vi "Broadcast D-O Settings.vi"(8 "error in (no error)":errorcluster, 10 "Message Queues":T7, 11 "D-O Module Config":T1={"GUID"="", "Drop Coords"={"Horizontal"=0, "Vertical"=0}, "Process Name"="", "User name"="", "Queue Name"="", "Settings"={"Valve Settings"={"D-O Settings"={"DAQmx Task Name"="", "Output Channel"=0, "Output Channel Names"=[]}, "VICI Electronic Actuator"={"VISA resource name"="", "Mode"=enum."Two Positions With Stops", "Simulated"=FALSE}}, "Valve Type"=enum."Digital Output Valve", "Time On (Sec)"=0.0, "Time Off (Sec)"=0.0, "Run?"=FALSE}, "Load Count"=0} {"Settings"."Valve Settings"."D-O Settings"."Output Channel" items=["Choose a Channel"]}) -> (0 "error out":errorcluster)   [LabVIEW 2018, in "D-O Module.lvlib"]
uses:
  D-O Module.lvlib
  All Message Queues.ctl
  support/Message Queue/Message Cluster.ctl
  D-O Module Config Cluster.ctl
  <vilib>/Utility/miscctls.llb/LVPoint32TypeDef.ctl
  Valve Clusters.ctl
  D-O Module Settings Cluster.ctl
  D-O Device Settings Cluster.ctl
  VICI Electronic Actuator/VICI Electronic Actuator Settings.ctl
  support/Message Queue/Enqueue Message (Single).vi
  support/Message Queue/Message Queue.lvlib
  Shared Variables/Dynamic Shared Variables.lvlib
  DIO Valve/VICI Electronic Actuator.lvlib
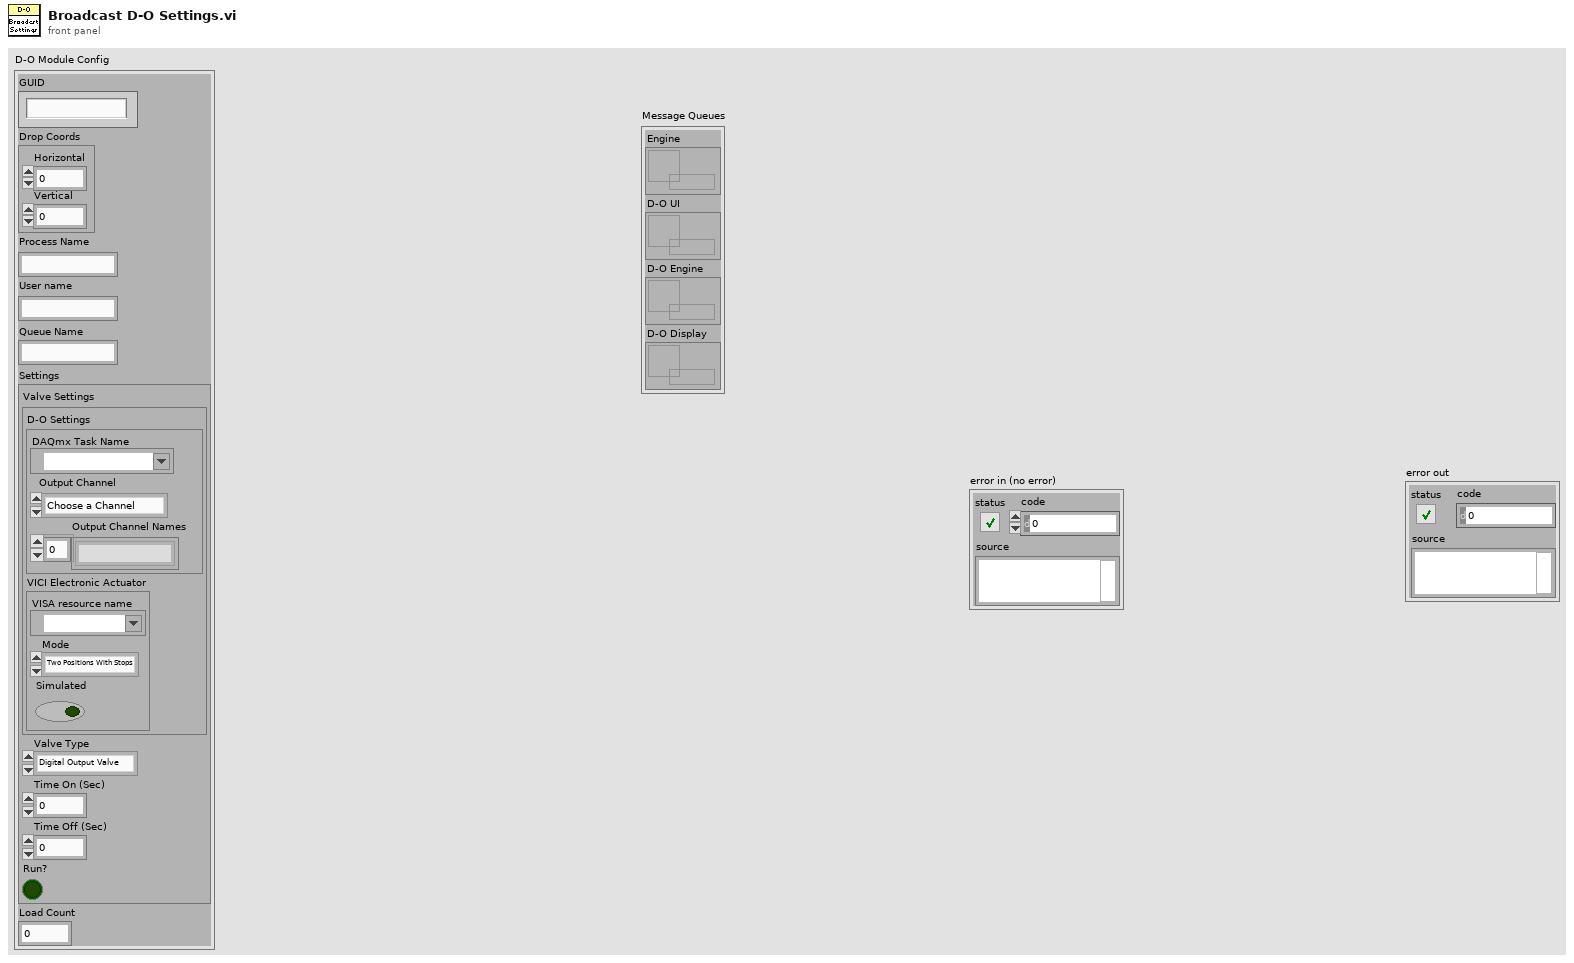
[diagram p1: front panel]
types:
  T1 = typedef "D-O Module.lvlib/D-O Module Config Cluster.ctl" = cluster{"GUID":string, "Drop Coords":T2, "Process Name":string, "User name":string, "Queue Name":string, "Settings":T3, "Load Count":i32}
  T2 = typedef "LVPoint32TypeDef.ctl" = cluster{"Horizontal":i32, "Vertical":i32}
  T3 = typedef "D-O Module.lvlib/Valve Clusters.ctl" = cluster{"Valve Settings":T4, "Valve Type":enum16{"Default", "Digital Output Valve", "VICI Electronic Actuator"}, "Time On (Sec)":dbl, "Time Off (Sec)":dbl, "Run?":bool}
  T4 = typedef "D-O Module.lvlib/D-O Module Settings Cluster.ctl" = cluster{"D-O Settings":T5, "VICI Electronic Actuator":T6}
  T5 = typedef "D-O Module.lvlib/D-O Device Settings Cluster.ctl" = cluster{"DAQmx Task Name":refnum<k21>, "Output Channel":u16, "Output Channel Names":string[]}
  T6 = typedef "VICI Electronic Actuator.lvlib/VICI Electronic Actuator Settings.ctl" = cluster{"VISA resource name":refnum<visa-resource-name>, "Mode":enum16{"Two Positions With Stops", "Two Positions Without Stops", "Mutiposition"}, "Simulated":bool}
  T7 = typedef "D-O Module.lvlib/All Message Queues.ctl" = cluster{"Engine":refnum<queue>, "D-O UI":refnum<queue>, "D-O Engine":refnum<queue>, "D-O Display":refnum<queue>}
  T8 = cluster{"enable? (F)":bool, "name":string, "alarm on":bool, "priority":u32, "ack type":enum16{"Auto", "User", "None", "Each Occurrence"}, "area":string, "description":string, "log? (T)":bool}
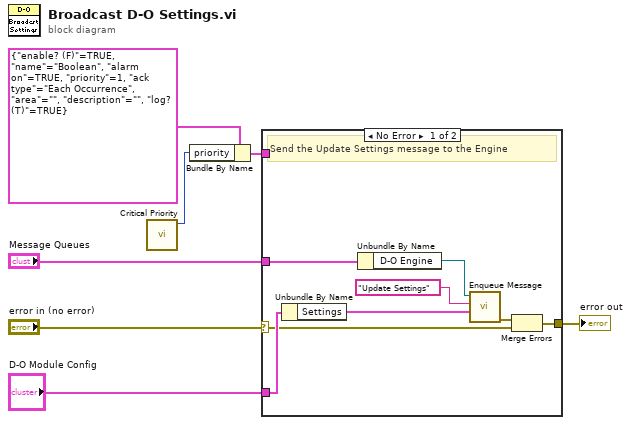
[diagram p0: block diagram]
diagram:
  n1 = call "Critical Priority.vi"() -> ("critical priority"=w3:i32)  [unwired: 11 in]
  n2 = Bundle By Name(cluster=T8 {"enable? (F)"=TRUE, "name"="Boolean", "alarm on"=TRUE, "priority"=1, "ack type"=enum."Each Occurrence", "area"="", "description"="", "log? (T)"=TRUE} ("Boolean alarm settings"), "priority"=w3) -> (w2:T8)
  n3 = case shown="No Error" "error in (no error)" {
    selector: "error in (no error)" -> [w13 w16]
    tunnel: [w15 w16] -> w5
    tunnel: "D-O Module Config" -> [w14 _]
    tunnel: "Message Queues" -> [w12 _]
    tunnel: w2 -> [_ _]
    frame No Error {
      # "Send the Update Settings message to the Engine"
      n4 = Unbundle By Name(w14) -> ("Settings"=w8:T3)
      n5 = Unbundle By Name(w12) -> ("D-O Engine"=w11:refnum<queue>)
      n6 = call-poly "Enqueue Message.vi"("Message Data"=w8, "Message"="Update Settings", "Message Queue"=w11) -> ("error out"=w10:errorcluster)  [unwired: 7 in, 1 out]
      n7 = Merge Errors(w10, w13) -> (w15:errorcluster)
    }
    frame Error {
    }
  }
  "error out" <- w5
